vi "大富翁.vi"() -> ()   [LabVIEW 2014] (continued)
                      n4719 = local read "位置 3"() -> (w3962:dbl)
                      n4720 = Increment(x=w3962) -> (x+1=w3961:dbl)
                      n4721 = local write "位置 3"(w3961) -> ()
                    }
                    frame 33..36 {
                      n4722 = property on="P3 棋子" class="Bool (strict)"() -> ("Top"=w3967:i32)  [unwired: 2 in, 2 out]
                      n4723 = Subtract(x=w3967, y=96) -> (x-y=w3968:i32)
                      n4724 = property on="P3 棋子" class="Bool (strict)"("Top"=w3968) -> ()  [unwired: 2 in, 2 out]
                      n4725 = Wait (ms)(milliseconds to wait=u32 700) -> ()  [unwired: 1 out]
                      n4726 = local read "位置 3"() -> (w3966:dbl)
                      n4727 = Increment(x=w3966) -> (x+1=w3965:dbl)
                      n4728 = local write "位置 3"(w3965) -> ()
                    }
                    frame 37 {
                      n4729 = property on="P3 棋子" class="Bool (strict)"("Top"=144 ("Position:Top")) -> ()  [unwired: 2 in, 2 out]
                      n4730 = Wait (ms)(milliseconds to wait=u32 700) -> ()  [unwired: 1 out]
                      n4731 = local write "位置 3"(0.0 ("位置 1")) -> ()
                    }
                  }
                }
              }
              frame #2 {
                n4732 = local read "位置 3"() -> (w3974:dbl)
              }
            }
          }
          frame 41 {
            n4733 = stacked-sequence {
              tunnel: [_ _ w4049] -> w3976
              frame #0 {
                w3977 = T1."Disabled" ("Disabled")
                n4734 = property on="擲骰子 4" class="Bool (strict)"("DisabledEnum"=w3977) -> ()  [unwired: 2 in, 2 out]
                n4735 = property on="擲骰子 2" class="Bool (strict)"("DisabledEnum"=w3977) -> ()  [unwired: 2 in, 2 out]
                n4736 = property on="擲骰子 3" class="Bool (strict)"("DisabledEnum"=w3977) -> ()  [unwired: 2 in, 2 out]
                n4737 = property on="擲骰子 1" class="Bool (strict)"("DisabledEnum"=w3977) -> ()  [unwired: 2 in, 2 out]
                n4738 = for {
                  N: 70 -> [_]
                  n4739 = call "dice.vi"() -> ("y"=w3980:dbl)  [unwired: 11 in]
                  n4740 = local write "骰子"(w3980) -> ()
                  n4741 = Wait (ms)(milliseconds to wait=u32 10) -> ()  [unwired: 1 out]
                }
                n4742 = local write "擲骰子 4"(FALSE ("擲骰子 4")) -> ()
              }
              frame #1 {
                n4743 = local read "骰子"() -> (w3982:dbl)
                n4744 = for {
                  N: w3982 -> [_]
                  i -> [w3984]
                  n4745 = local read "位置 4"() -> (w3983:dbl)
                  n4746 = case shown="0" w3983 {
                    tunnel: w3984 -> [w3986 _ _ _ _ _ _ _ _ _ _ _]
                    frame 0 {
                      n4747 = Greater Than 0?(x=w3986) -> (x > 0?=w3985:bool)
                      n4748 = case shown="True" w3985 {
                        frame False {
                          n4749 = property on="P4 棋子" class="Bool (strict)"("Left"=337 ("Position:Left")) -> ()  [unwired: 2 in, 2 out]
                          n4750 = Wait (ms)(milliseconds to wait=u32 700) -> ()  [unwired: 1 out]
                          n4751 = local read "位置 4"() -> (w3989:dbl)
                          n4752 = Increment(x=w3989) -> (x+1=w3988:dbl)
                          n4753 = local write "位置 4"(w3988) -> ()
                        }
                        frame True {
                          n4754 = property on="P4 棋子" class="Bool (strict)"("Left"=337 ("Position:Left")) -> ()  [unwired: 2 in, 2 out]
                          n4755 = Wait (ms)(milliseconds to wait=u32 700) -> ()  [unwired: 1 out]
                          n4756 = local read "玩家四財產"() -> (w3992:dbl)
                          n4757 = local read "位置 4"() -> (w3994:dbl)
                          n4758 = Add(x=w3992, y=2000.0) -> (x+y=w3991:dbl)
                          n4759 = Increment(x=w3994) -> (x+1=w3993:dbl)
                          n4760 = local write "位置 4"(w3993) -> ()
                          n4761 = local write "玩家四財產"(w3991) -> ()
                        }
                      }
                    }
                    frame 1..11, Default {
                      n4762 = property on="P4 棋子" class="Bool (strict)"() -> ("Left"=w4000:i32)  [unwired: 2 in, 2 out]
                      n4763 = Add(x=w4000, y=96) -> (x+y=w4001:i32)
                      n4764 = property on="P4 棋子" class="Bool (strict)"("Left"=w4001) -> ()  [unwired: 2 in, 2 out]
                      n4765 = Wait (ms)(milliseconds to wait=u32 700) -> ()  [unwired: 1 out]
                      n4766 = local read "位置 4"() -> (w3999:dbl)
                      n4767 = Increment(x=w3999) -> (x+1=w3998:dbl)
                      n4768 = local write "位置 4"(w3998) -> ()
                    }
                    frame 12 {
                      n4769 = property on="P4 棋子" class="Bool (strict)"("Left"=1540 ("Position:Left")) -> ()  [unwired: 2 in, 2 out]
                      n4770 = Wait (ms)(milliseconds to wait=u32 700) -> ()  [unwired: 1 out]
                      n4771 = local read "位置 4"() -> (w4005:dbl)
                      n4772 = Increment(x=w4005) -> (x+1=w4004:dbl)
                      n4773 = local write "位置 4"(w4004) -> ()
                    }
                    frame 13 {
                      n4774 = property on="P4 棋子" class="Bool (strict)"("Top"=275 ("Position:Top")) -> ()  [unwired: 2 in, 2 out]
                      n4775 = Wait (ms)(milliseconds to wait=u32 700) -> ()  [unwired: 1 out]
                      n4776 = local read "位置 4"() -> (w4009:dbl)
                      n4777 = Increment(x=w4009) -> (x+1=w4008:dbl)
                      n4778 = local write "位置 4"(w4008) -> ()
                    }
                    frame 14..17 {
                      n4779 = property on="P4 棋子" class="Bool (strict)"() -> ("Top"=w4014:i32)  [unwired: 2 in, 2 out]
                      n4780 = Add(x=w4014, y=96) -> (x+y=w4015:i32)
                      n4781 = property on="P4 棋子" class="Bool (strict)"("Top"=w4015) -> ()  [unwired: 2 in, 2 out]
                      n4782 = Wait (ms)(milliseconds to wait=u32 700) -> ()  [unwired: 1 out]
                      n4783 = local read "位置 4"() -> (w4013:dbl)
                      n4784 = Increment(x=w4013) -> (x+1=w4012:dbl)
                      n4785 = local write "位置 4"(w4012) -> ()
                    }
                    frame 18 {
                      n4786 = property on="P4 棋子" class="Bool (strict)"("Top"=798 ("Position:Top")) -> ()  [unwired: 2 in, 2 out]
                      n4787 = Wait (ms)(milliseconds to wait=u32 700) -> ()  [unwired: 1 out]
                      n4788 = local read "位置 4"() -> (w4019:dbl)
                      n4789 = Increment(x=w4019) -> (x+1=w4018:dbl)
                      n4790 = local write "位置 4"(w4018) -> ()
                    }
                    frame 19 {
                      n4791 = property on="P4 棋子" class="Bool (strict)"("Left"=1393 ("Position:Top")) -> ()  [unwired: 2 in, 2 out]
                      n4792 = Wait (ms)(milliseconds to wait=u32 700) -> ()  [unwired: 1 out]
                      n4793 = local read "位置 4"() -> (w4023:dbl)
                      n4794 = Increment(x=w4023) -> (x+1=w4022:dbl)
                      n4795 = local write "位置 4"(w4022) -> ()
                    }
                    frame 20..30 {
                      n4796 = property on="P4 棋子" class="Bool (strict)"() -> ("Left"=w4028:i32)  [unwired: 2 in, 2 out]
                      n4797 = Subtract(x=w4028, y=96) -> (x-y=w4029:i32)
                      n4798 = property on="P4 棋子" class="Bool (strict)"("Left"=w4029) -> ()  [unwired: 2 in, 2 out]
                      n4799 = Wait (ms)(milliseconds to wait=u32 700) -> ()  [unwired: 1 out]
                      n4800 = local read "位置 4"() -> (w4027:dbl)
                      n4801 = Increment(x=w4027) -> (x+1=w4026:dbl)
                      n4802 = local write "位置 4"(w4026) -> ()
                    }
                    frame 31 {
                      n4803 = property on="P4 棋子" class="Bool (strict)"("Left"=197 ("Position:Top")) -> ()  [unwired: 2 in, 2 out]
                      n4804 = Wait (ms)(milliseconds to wait=u32 700) -> ()  [unwired: 1 out]
                      n4805 = local read "位置 4"() -> (w4033:dbl)
                      n4806 = Increment(x=w4033) -> (x+1=w4032:dbl)
                      n4807 = local write "位置 4"(w4032) -> ()
                    }
                    frame 32 {
                      n4808 = property on="P4 棋子" class="Bool (strict)"("Top"=659 ("Position:Top")) -> ()  [unwired: 2 in, 2 out]
                      n4809 = Wait (ms)(milliseconds to wait=u32 700) -> ()  [unwired: 1 out]
                      n4810 = local read "位置 4"() -> (w4037:dbl)
                      n4811 = Increment(x=w4037) -> (x+1=w4036:dbl)
                      n4812 = local write "位置 4"(w4036) -> ()
                    }
                    frame 33..36 {
                      n4813 = property on="P4 棋子" class="Bool (strict)"() -> ("Top"=w4042:i32)  [unwired: 2 in, 2 out]
                      n4814 = Subtract(x=w4042, y=96) -> (x-y=w4043:i32)
                      n4815 = property on="P4 棋子" class="Bool (strict)"("Top"=w4043) -> ()  [unwired: 2 in, 2 out]
                      n4816 = Wait (ms)(milliseconds to wait=u32 700) -> ()  [unwired: 1 out]
                      n4817 = local read "位置 4"() -> (w4041:dbl)
                      n4818 = Increment(x=w4041) -> (x+1=w4040:dbl)
                      n4819 = local write "位置 4"(w4040) -> ()
                    }
                    frame 37 {
                      n4820 = property on="P4 棋子" class="Bool (strict)"("Top"=144 ("Position:Top")) -> ()  [unwired: 2 in, 2 out]
                      n4821 = Wait (ms)(milliseconds to wait=u32 700) -> ()  [unwired: 1 out]
                      n4822 = local write "位置 4"(0.0 ("位置 4")) -> ()
                    }
                  }
                }
              }
              frame #2 {
                n4823 = local read "位置 4"() -> (w4049:dbl)
              }
            }
          }
          frame 42 {
            n4824 = local read "遊戲人數"() -> (w4052:dbl)
            n4825 = case shown="2, Default" w4052 {
              tunnel: [w4053 w4090 w4145] -> w4051
              frame 2, Default {
                # "兩人"
                n4826 = local read "換誰?"() -> (w4054:dbl)
                n4827 = case shown="1, Default" w4054 {
                  tunnel: [w4056 w4073] -> w4053
                  frame 1, Default {
                    # "1回合結束"
                    n4828 = local read "剩幾天 2"() -> (w4059:dbl)
                    n4829 = Greater?(x=w4059, y=0.0) -> (0:w4057:bool)
                    n4830 = case shown="True" w4057 {
                      tunnel: [-100 42] -> w4056
                      frame False {
                        # "換2回合"
                        n4831 = property on="擲骰子 1" class="Bool (strict)"("Visible"=FALSE) -> ()  [unwired: 2 in, 2 out]
                        n4832 = property on="擲骰子 2" class="Bool (strict)"("DisabledEnum"=T1."Enabled" ("Disabled")) -> ()  [unwired: 2 in, 2 out]
                        n4833 = property on="擲骰子 2" class="Bool (strict)"("Visible"=TRUE) -> ()  [unwired: 2 in, 2 out]
                      }
                      frame True {
                        # "2坐牢"
                        n4834 = stacked-sequence {
                          frame #0 {
                            n4835 = local write "擲骰子 1"(FALSE ("擲骰子 1")) -> ()
                            n4836 = property on="擲骰子 1" class="Bool (strict)"("Visible"=FALSE) -> ()  [unwired: 2 in, 2 out]
                          }
                          frame #1 {
                            n4837 = local read "剩幾天 2"() -> (w4067:dbl)
                            n4838 = property on="擲骰子 2" class="Bool (strict)"("Visible"=TRUE) -> ()  [unwired: 2 in, 2 out]
                            n4839 = call "入獄還有幾天.vi"("過路費"=w4067) -> ()  [unwired: 3 in]
                            n4840 = property on="擲骰子 2" class="Bool (strict)"("DisabledEnum"=T1."Disabled and Grayed Out" ("Disabled")) -> ()  [unwired: 2 in, 2 out]
                          }
                          frame #2 {
                            n4841 = local read "剩幾天 2"() -> (w4071:dbl)
                            n4842 = Decrement(x=w4071) -> (x-1=w4070:dbl)
                            n4843 = case shown="1, Default" w4070 {
                              frame 0 {
                                n4844 = property on="入獄 2" class="Bool (strict)"("Visible"=FALSE) -> ()  [unwired: 2 in, 2 out]
                              }
                              frame 1, Default {
                              }
                            }
                            n4845 = local write "剩幾天 2"(w4070) -> ()
                          }
                        }
                      }
                    }
                    n4846 = local write "換誰?"(2.0 ("換誰?")) -> ()
                  }
                  frame 2 {
                    # "2回合結束"
                    n4847 = local read "剩幾天 1"() -> (w4074:dbl)
                    n4848 = Greater?(x=w4074, y=0.0) -> (0:w4076:bool)
                    n4849 = case shown="False" w4076 {
                      tunnel: [-100 42] -> w4073
                      frame False {
                        # "換1回合"
                        n4850 = property on="擲骰子 1" class="Bool (strict)"("Visible"=TRUE) -> ()  [unwired: 2 in, 2 out]
                        n4851 = property on="擲骰子 2" class="Bool (strict)"("Visible"=FALSE) -> ()  [unwired: 2 in, 2 out]
                        n4852 = property on="擲骰子 1" class="Bool (strict)"("DisabledEnum"=T1."Enabled" ("Disabled")) -> ()  [unwired: 2 in, 2 out]
                      }
                      frame True {
                        # "1坐牢"
                        n4853 = stacked-sequence {
                          frame #0 {
                            n4854 = property on="擲骰子 2" class="Bool (strict)"("Visible"=FALSE) -> ()  [unwired: 2 in, 2 out]
                          }
                          frame #1 {
                            n4855 = local read "剩幾天 1"() -> (w4084:dbl)
                            n4856 = call "入獄還有幾天.vi"("過路費"=w4084) -> ()  [unwired: 3 in]
                            n4857 = property on="擲骰子 1" class="Bool (strict)"("Visible"=TRUE) -> ()  [unwired: 2 in, 2 out]
                            n4858 = property on="擲骰子 1" class="Bool (strict)"("DisabledEnum"=T1."Disabled and Grayed Out" ("Disabled")) -> ()  [unwired: 2 in, 2 out]
                          }
                          frame #2 {
                            n4859 = local read "剩幾天 1"() -> (w4088:dbl)
                            n4860 = Decrement(x=w4088) -> (x-1=w4087:dbl)
                            n4861 = case shown="0" w4087 {
                              frame 0 {
                                n4862 = property on="入獄 1" class="Bool (strict)"("Visible"=FALSE) -> ()  [unwired: 2 in, 2 out]
                              }
                              frame 1, Default {
                              }
                            }
                            n4863 = local write "剩幾天 1"(w4087) -> ()
                          }
                        }
                      }
                    }
                    n4864 = local write "換誰?"(1.0 ("換誰?")) -> ()
                  }
                }
              }
              frame 3 {
                # "三人"
                n4865 = local read "換誰?"() -> (w4091:dbl)
                n4866 = case shown="3" w4091 {
                  tunnel: [w4093 w4111 w4127] -> w4090
                  frame 1, Default {
                    # "1回合結束"
                    n4867 = local read "剩幾天 2"() -> (w4096:dbl)
                    n4868 = local write "換誰?"(2.0 ("換誰?")) -> ()
                    n4869 = Greater?(x=w4096, y=0.0) -> (0:w4094:bool)
                    n4870 = case shown="False" w4094 {
                      tunnel: [-100 42] -> w4093
                      frame False {
                        # "換2回合"
                        n4871 = property on="擲骰子 1" class="Bool (strict)"("Visible"=FALSE) -> ()  [unwired: 2 in, 2 out]
                        n4872 = property on="擲骰子 2" class="Bool (strict)"("DisabledEnum"=T1."Enabled" ("Disabled")) -> ()  [unwired: 2 in, 2 out]
                        n4873 = property on="擲骰子 2" class="Bool (strict)"("Visible"=TRUE) -> ()  [unwired: 2 in, 2 out]
                      }
                      frame True {
                        # "2坐牢"
                        n4874 = stacked-sequence {
                          frame #0 {
                            n4875 = local write "擲骰子 1"(FALSE ("擲骰子 1")) -> ()
                            n4876 = property on="擲骰子 1" class="Bool (strict)"("Visible"=FALSE) -> ()  [unwired: 2 in, 2 out]
                          }
                          frame #1 {
                            n4877 = local read "剩幾天 2"() -> (w4104:dbl)
                            n4878 = property on="擲骰子 2" class="Bool (strict)"("Visible"=TRUE) -> ()  [unwired: 2 in, 2 out]
                            n4879 = call "入獄還有幾天.vi"("過路費"=w4104) -> ()  [unwired: 3 in]
                            n4880 = property on="擲骰子 2" class="Bool (strict)"("DisabledEnum"=T1."Disabled and Grayed Out" ("Disabled")) -> ()  [unwired: 2 in, 2 out]
                          }
                          frame #2 {
                            n4881 = local read "剩幾天 2"() -> (w4108:dbl)
                            n4882 = Decrement(x=w4108) -> (x-1=w4107:dbl)
                            n4883 = case shown="0" w4107 {
                              frame 0 {
                                n4884 = property on="入獄 2" class="Bool (strict)"("Visible"=FALSE) -> ()  [unwired: 2 in, 2 out]
                              }
                              frame 1, Default {
                              }
                            }
                            n4885 = local write "剩幾天 2"(w4107) -> ()
                          }
                        }
                      }
                    }
                  }
                  frame 2 {
                    # "2回合結束"
                    n4886 = local read "剩幾天 3"() -> (w4110:dbl)
                    n4887 = local write "換誰?"(3.0 ("換誰?")) -> ()
                    n4888 = Greater?(x=w4110, y=0.0) -> (0:w4113:bool)
                    n4889 = case shown="False" w4113 {
                      tunnel: [-100 42] -> w4111
                      frame False {
                        # "換3回合"
                        n4890 = property on="擲骰子 2" class="Bool (strict)"("Visible"=FALSE) -> ()  [unwired: 2 in, 2 out]
                        n4891 = property on="擲骰子 3" class="Bool (strict)"("Visible"=TRUE) -> ()  [unwired: 2 in, 2 out]
                        n4892 = property on="擲骰子 3" class="Bool (strict)"("DisabledEnum"=T1."Enabled" ("Disabled")) -> ()  [unwired: 2 in, 2 out]
                      }
                      frame True {
                        # "3坐牢"
                        n4893 = stacked-sequence {
                          frame #0 {
                            n4894 = property on="擲骰子 2" class="Bool (strict)"("Visible"=FALSE) -> ()  [unwired: 2 in, 2 out]
                          }
                          frame #1 {
                            n4895 = local read "剩幾天 3"() -> (w4121:dbl)
                            n4896 = call "入獄還有幾天.vi"("過路費"=w4121) -> ()  [unwired: 3 in]
                            n4897 = property on="擲骰子 3" class="Bool (strict)"("DisabledEnum"=T1."Disabled and Grayed Out" ("Disabled")) -> ()  [unwired: 2 in, 2 out]
                            n4898 = property on="擲骰子 3" class="Bool (strict)"("Visible"=TRUE) -> ()  [unwired: 2 in, 2 out]
                          }
                          frame #2 {
                            n4899 = local read "剩幾天 3"() -> (w4125:dbl)
                            n4900 = Decrement(x=w4125) -> (x-1=w4124:dbl)
                            n4901 = case shown="0" w4124 {
                              frame 0 {
                                n4902 = property on="入獄 3" class="Bool (strict)"("Visible"=FALSE) -> ()  [unwired: 2 in, 2 out]
                              }
                              frame 1, Default {
                              }
                            }
                            n4903 = local write "剩幾天 3"(w4124) -> ()
                          }
                        }
                      }
                    }
                  }
                  frame 3 {
                    # "3回合結束"
                    n4904 = local read "剩幾天 1"() -> (w4128:dbl)
                    n4905 = local write "換誰?"(1.0 ("換誰?")) -> ()
                    n4906 = Greater?(x=w4128, y=0.0) -> (0:w4130:bool)
                    n4907 = case shown="False" w4130 {
                      tunnel: [-100 42] -> w4127
                      frame False {
                        # "換1回合"
                        n4908 = property on="擲骰子 1" class="Bool (strict)"("Visible"=TRUE) -> ()  [unwired: 2 in, 2 out]
                        n4909 = property on="擲骰子 2" class="Bool (strict)"("Visible"=FALSE) -> ()  [unwired: 2 in, 2 out]
                        n4910 = property on="擲骰子 1" class="Bool (strict)"("DisabledEnum"=T1."Enabled" ("Disabled")) -> ()  [unwired: 2 in, 2 out]
                        n4911 = property on="擲骰子 3" class="Bool (strict)"("Visible"=FALSE) -> ()  [unwired: 2 in, 2 out]
                      }
                      frame True {
                        # "1坐牢"
                        n4912 = stacked-sequence {
                          frame #0 {
                            n4913 = property on="擲骰子 3" class="Bool (strict)"("Visible"=FALSE) -> ()  [unwired: 2 in, 2 out]
                          }
                          frame #1 {
                            n4914 = local read "剩幾天 1"() -> (w4139:dbl)
                            n4915 = call "入獄還有幾天.vi"("過路費"=w4139) -> ()  [unwired: 3 in]
                            n4916 = property on="擲骰子 1" class="Bool (strict)"("Visible"=TRUE) -> ()  [unwired: 2 in, 2 out]
                            n4917 = property on="擲骰子 1" class="Bool (strict)"("DisabledEnum"=T1."Disabled and Grayed Out" ("Disabled")) -> ()  [unwired: 2 in, 2 out]
                          }
                          frame #2 {
                            n4918 = local read "剩幾天 1"() -> (w4143:dbl)
                            n4919 = Decrement(x=w4143) -> (x-1=w4142:dbl)
                            n4920 = case shown="0" w4142 {
                              frame 0 {
                                n4921 = property on="入獄 1" class="Bool (strict)"("Visible"=FALSE) -> ()  [unwired: 2 in, 2 out]
                              }
                              frame 1, Default {
                              }
                            }
                            n4922 = local write "剩幾天 1"(w4142) -> ()
                          }
                        }
                      }
                    }
                  }
                }
              }
              frame 4 {
                # "四人"
                n4923 = local read "換誰?"() -> (w4146:dbl)
                n4924 = case shown="1, Default" w4146 {
                  tunnel: [w4148 w4166 w4183 w4201] -> w4145
                  frame 1, Default {
                    # "1回合結束"
                    n4925 = local read "剩幾天 2"() -> (w4151:dbl)
                    n4926 = local write "換誰?"(2.0 ("換誰?")) -> ()
                    n4927 = Greater?(x=w4151, y=0.0) -> (0:w4149:bool)
                    n4928 = case shown="False" w4149 {
                      tunnel: [-100 42] -> w4148
                      frame False {
                        # "換2回合"
                        n4929 = property on="擲骰子 1" class="Bool (strict)"("Visible"=FALSE) -> ()  [unwired: 2 in, 2 out]
                        n4930 = property on="擲骰子 2" class="Bool (strict)"("DisabledEnum"=T1."Enabled" ("Disabled")) -> ()  [unwired: 2 in, 2 out]
                        n4931 = property on="擲骰子 2" class="Bool (strict)"("Visible"=TRUE) -> ()  [unwired: 2 in, 2 out]
                      }
                      frame True {
                        # "2坐牢"
                        n4932 = stacked-sequence {
                          frame #0 {
                            n4933 = local write "擲骰子 1"(FALSE ("擲骰子 1")) -> ()
                            n4934 = property on="擲骰子 1" class="Bool (strict)"("Visible"=FALSE) -> ()  [unwired: 2 in, 2 out]
                          }
                          frame #1 {
                            n4935 = local read "剩幾天 2"() -> (w4159:dbl)
                            n4936 = property on="擲骰子 2" class="Bool (strict)"("Visible"=TRUE) -> ()  [unwired: 2 in, 2 out]
                            n4937 = call "入獄還有幾天.vi"("過路費"=w4159) -> ()  [unwired: 3 in]
                            n4938 = property on="擲骰子 2" class="Bool (strict)"("DisabledEnum"=T1."Disabled and Grayed Out" ("Disabled")) -> ()  [unwired: 2 in, 2 out]
                          }
                          frame #2 {
                            n4939 = local read "剩幾天 2"() -> (w4163:dbl)
                            n4940 = Decrement(x=w4163) -> (x-1=w4162:dbl)
                            n4941 = case shown="0" w4162 {
                              frame 0 {
                                n4942 = property on="入獄 2" class="Bool (strict)"("Visible"=FALSE) -> ()  [unwired: 2 in, 2 out]
                              }
                              frame 1, Default {
                              }
                            }
                            n4943 = local write "剩幾天 2"(w4162) -> ()
                          }
                        }
                      }
                    }
                  }
                  frame 2 {
                    # "2回合結束"
                    n4944 = local read "剩幾天 3"() -> (w4165:dbl)
                    n4945 = local write "換誰?"(3.0 ("換誰?")) -> ()
                    n4946 = Greater?(x=w4165, y=0.0) -> (0:w4168:bool)
                    n4947 = case shown="False" w4168 {
                      tunnel: [-100 42] -> w4166
                      frame False {
                        # "換3回合"
                        n4948 = property on="擲骰子 2" class="Bool (strict)"("Visible"=FALSE) -> ()  [unwired: 2 in, 2 out]
                        n4949 = property on="擲骰子 3" class="Bool (strict)"("Visible"=TRUE) -> ()  [unwired: 2 in, 2 out]
                        n4950 = property on="擲骰子 3" class="Bool (strict)"("DisabledEnum"=T1."Enabled" ("Disabled")) -> ()  [unwired: 2 in, 2 out]
                      }
                      frame True {
                        # "3坐牢"
                        n4951 = stacked-sequence {
                          frame #0 {
                            n4952 = property on="擲骰子 2" class="Bool (strict)"("Visible"=FALSE) -> ()  [unwired: 2 in, 2 out]
                          }
                          frame #1 {
                            n4953 = local read "剩幾天 3"() -> (w4176:dbl)
                            n4954 = call "入獄還有幾天.vi"("過路費"=w4176) -> ()  [unwired: 3 in]
                            n4955 = property on="擲骰子 3" class="Bool (strict)"("DisabledEnum"=T1."Disabled and Grayed Out" ("Disabled")) -> ()  [unwired: 2 in, 2 out]
                            n4956 = property on="擲骰子 3" class="Bool (strict)"("Visible"=TRUE) -> ()  [unwired: 2 in, 2 out]
                          }
                          frame #2 {
                            n4957 = local read "剩幾天 3"() -> (w4180:dbl)
                            n4958 = Decrement(x=w4180) -> (x-1=w4179:dbl)
                            n4959 = case shown="0" w4179 {
                              frame 0 {
                                n4960 = property on="入獄 3" class="Bool (strict)"("Visible"=FALSE) -> ()  [unwired: 2 in, 2 out]
                              }
                              frame 1, Default {
                              }
                            }
                            n4961 = local write "剩幾天 3"(w4179) -> ()
                          }
                        }
                      }
                    }
                  }
                  frame 3 {
                    # "3回合結束"
                    n4962 = local read "剩幾天 4"() -> (w4182:dbl)
                    n4963 = local write "換誰?"(4.0 ("換誰?")) -> ()
                    n4964 = Greater?(x=w4182, y=0.0) -> (0:w4185:bool)
                    n4965 = case shown="False" w4185 {
                      tunnel: [-100 42] -> w4183
                      frame False {
                        # "換4回合"
                        n4966 = property on="擲骰子 1" class="Bool (strict)"("Visible"=FALSE) -> ()  [unwired: 2 in, 2 out]
                        n4967 = property on="擲骰子 2" class="Bool (strict)"("Visible"=FALSE) -> ()  [unwired: 2 in, 2 out]
                        n4968 = property on="擲骰子 3" class="Bool (strict)"("Visible"=FALSE) -> ()  [unwired: 2 in, 2 out]
                        n4969 = property on="擲骰子 4" class="Bool (strict)"("Visible"=TRUE) -> ()  [unwired: 2 in, 2 out]
                        n4970 = property on="擲骰子 4" class="Bool (strict)"("DisabledEnum"=T1."Enabled" ("Disabled")) -> ()  [unwired: 2 in, 2 out]
                      }
                      frame True {
                        # "4坐牢"
                        n4971 = stacked-sequence {
                          frame #0 {
                            n4972 = property on="擲骰子 3" class="Bool (strict)"("Visible"=FALSE) -> ()  [unwired: 2 in, 2 out]
                          }
                          frame #1 {
                            n4973 = local read "剩幾天 4"() -> (w4195:dbl)
                            n4974 = call "入獄還有幾天.vi"("過路費"=w4195) -> ()  [unwired: 3 in]
                            n4975 = property on="擲骰子 4" class="Bool (strict)"("Visible"=TRUE) -> ()  [unwired: 2 in, 2 out]
                            n4976 = property on="擲骰子 4" class="Bool (strict)"("DisabledEnum"=T1."Disabled and Grayed Out" ("Disabled")) -> ()  [unwired: 2 in, 2 out]
                          }
                          frame #2 {
                            n4977 = local read "剩幾天 4"() -> (w4199:dbl)
                            n4978 = Decrement(x=w4199) -> (x-1=w4198:dbl)
                            n4979 = case shown="0" w4198 {
                              frame 0 {
                                n4980 = property on="入獄 4" class="Bool (strict)"("Visible"=FALSE) -> ()  [unwired: 2 in, 2 out]
                              }
                              frame 1, Default {
                              }
                            }
                            n4981 = local write "剩幾天 4"(w4198) -> ()
                          }
                        }
                      }
                    }
                  }
                  frame 4 {
                    # "4回合結束"
                    n4982 = local read "剩幾天 1"() -> (w4202:dbl)
                    n4983 = local write "換誰?"(1.0 ("換誰?")) -> ()
                    n4984 = Greater?(x=w4202, y=0.0) -> (0:w4204:bool)
                    n4985 = case shown="False" w4204 {
                      tunnel: [-100 42] -> w4201
                      frame False {
                        # "換1回合"
                        n4986 = property on="擲骰子 1" class="Bool (strict)"("Visible"=TRUE) -> ()  [unwired: 2 in, 2 out]
                        n4987 = property on="擲骰子 2" class="Bool (strict)"("Visible"=FALSE) -> ()  [unwired: 2 in, 2 out]
                        n4988 = property on="擲骰子 1" class="Bool (strict)"("DisabledEnum"=T1."Enabled" ("Disabled")) -> ()  [unwired: 2 in, 2 out]
                        n4989 = property on="擲骰子 3" class="Bool (strict)"("Visible"=FALSE) -> ()  [unwired: 2 in, 2 out]
                        n4990 = property on="擲骰子 4" class="Bool (strict)"("Visible"=FALSE) -> ()  [unwired: 2 in, 2 out]
                      }
                      frame True {
                        # "1坐牢"
                        n4991 = stacked-sequence {
                          frame #0 {
                            n4992 = property on="擲骰子 4" class="Bool (strict)"("Visible"=FALSE) -> ()  [unwired: 2 in, 2 out]
                          }
                          frame #1 {
                            n4993 = local read "剩幾天 1"() -> (w4214:dbl)
                            n4994 = call "入獄還有幾天.vi"("過路費"=w4214) -> ()  [unwired: 3 in]
                            n4995 = property on="擲骰子 1" class="Bool (strict)"("Visible"=TRUE) -> ()  [unwired: 2 in, 2 out]
                            n4996 = property on="擲骰子 1" class="Bool (strict)"("DisabledEnum"=T1."Disabled and Grayed Out" ("Disabled")) -> ()  [unwired: 2 in, 2 out]
                          }
                          frame #2 {
                            n4997 = local read "剩幾天 1"() -> (w4218:dbl)
                            n4998 = Decrement(x=w4218) -> (x-1=w4217:dbl)
                            n4999 = case shown="0" w4217 {
                              frame 0 {
                                n5000 = property on="入獄 1" class="Bool (strict)"("Visible"=FALSE) -> ()  [unwired: 2 in, 2 out]
                              }
                              frame 1, Default {
                              }
                            }
                            n5001 = local write "剩幾天 1"(w4217) -> ()
                          }
                        }
                      }
                    }
                  }
                }
              }
            }
          }
        }
      }
    }
  }
